vi "Run In UI.vi"(11 "LUnit Test Case in":refnum<class "LUnit Test Case.lvclass">) -> (3 "LUnit Test Case out":refnum<class "LUnit Test Case.lvclass">)   [LabVIEW 2020, in "LUnit Test Case.lvclass"]
uses:
  LUnit Test Case.lvclass
  LUnit Test Case.lvclass/LUnit Test Case.ctl
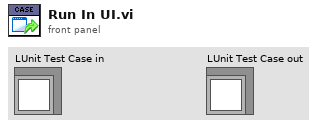
[diagram p1: front panel]
types:
  T1 = enum32{"Invalid", "Standard", "Closed", "Hidden", "Minimized", "Maximized"}
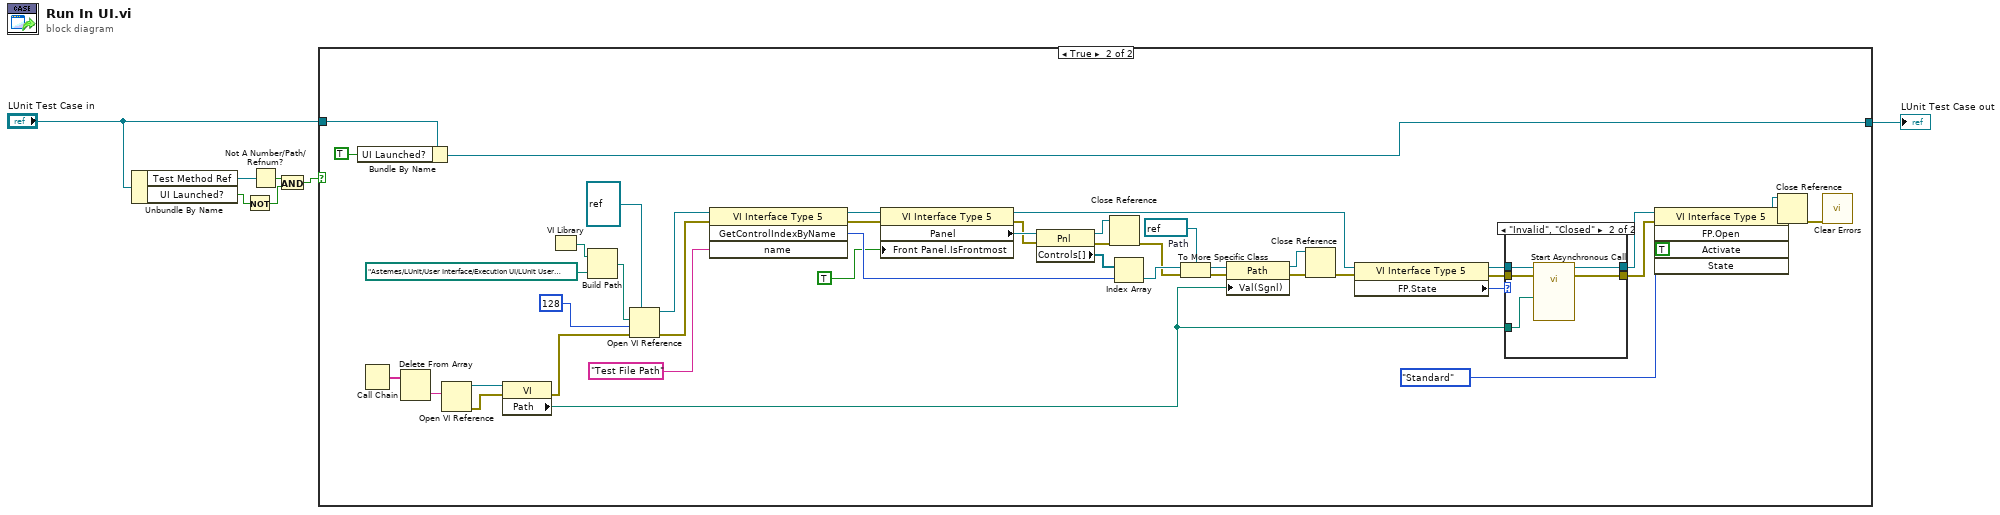
[diagram p0: block diagram]
diagram:
  n1 = Unbundle By Name("LUnit Test Case in") -> ("Test Method Ref"=w7:refnum<vi>, "UI Launched?"=w4:bool)
  n2 = Not(x=w4) -> (.not. x?=w3:bool)
  n3 = Not A Number/Path/Refnum?(number/path/refnum=w7) -> (NaN/Path/Refnum?=w6:bool)
  n4 = And(x=w6, y=w3) -> (x .and. y?=w5:bool)
  n5 = case shown="True" w5 {
    tunnel: "LUnit Test Case in" -> [w8 w11]
    tunnel: [w8 w9] -> w1
    frame False {
    }
    frame True {
      w40 = refnum<vi> refnum  # Path
      n6 = Bundle By Name(cluster=w11, "UI Launched?"=TRUE) -> (w9:refnum<class "LUnit Test Case.lvclass">)
      n7 = Call Chain() -> (call chain=w13:string[])
      n8 = Delete From Array(array=w13) -> (deleted portion=w17:string)  [unwired: 2 in, 1 out]
      n9 = Open VI Reference(vi path=w17) -> (vi reference=w16:refnum<vi>, error out=w14:errorcluster)  [unwired: 5 in]
      n10 = property class="VI"(reference=w16, error in=w14) -> (error out=w15:errorcluster, "Path"=w12:path)  [unwired: 1 out]
      n11 = VI Library() -> (path=w46:path)
      n12 = Build Path(base path=w46, name or relative path=path "Astemes/LUnit/User Interface/Execution UI/LUnit User Interface.vi" ("Relative Path from 1 to 2")) -> (appended path=w51:path)
      n13 = Open VI Reference(type specifier VI Refnum (for type only)=refnum<vi> refnum, vi path=w51, options=128, error in (no error)=w15) -> (vi reference=w28:refnum<vi>, error out=w27:errorcluster)  [unwired: 2 in]
      n14 = invoke class="VI Interface Type 5" method="GetControlIndexByName"(reference=w28, error in=w27, "name"="Test File Path" ("Control Name")) -> (reference out=w44:refnum<vi>, error out=w34:errorcluster, "GetControlIndexByName"=w41:i32)  [unwired: 1 in, 1 out]
      n15 = property class="VI Interface Type 5"(reference=w44, error in=w34, "Front Panel.IsFrontmost"=TRUE ("Front Panel Window:Is Frontmost")) -> (reference out=w21:refnum<vi>, error out=w35:errorcluster, "Panel"=w45:refnum<vi>)
      n16 = property class="Pnl"(reference=w45, error in=w35) -> (reference out=w31:refnum<vi>, error out=w36:errorcluster, "Controls[]"=w42:refnum<vi>[])
      n17 = Close Reference(reference=w31, error in (no error)=w36) -> (error out=w32:errorcluster)
      n18 = Index Array(array=w42, index=w41) -> (element=w38:refnum<vi>)
      n19 = To More Specific Class(target class=w40, reference=w38, error in=w32) -> (specific class reference=w39:refnum<vi>, error out=w37:errorcluster)
      n20 = property class="Path"(reference=w39, error in=w37, "Val(Sgnl)"=w12) -> (reference out=w30:refnum<vi>, error out=w33:errorcluster)
      n21 = Close Reference(reference=w30, error in (no error)=w33) -> (error out=w23:errorcluster)
      n22 = property class="VI Interface Type 5"(reference=w21, error in=w23) -> (reference out=w25:refnum<vi>, error out=w26:errorcluster, "FP.State"=w24:T1)
      n23 = case shown="\"Invalid\", \"Closed\"" w24 {
        tunnel: w26 -> [w55 w60]
        tunnel: w25 -> [w54 w59]
        tunnel: [w55 w57] -> w22
        tunnel: [w54 w58] -> w20
        tunnel: w12 -> [_ w56]
        frame Default {
        }
        frame "Invalid", "Closed" {
          n24 = call-by-ref "Start Asynchronous Call"(reference=w59, error in=w60, "Test File Path"=w56) -> (reference out=w58:refnum<vi>, error out=w57:errorcluster)  [unwired: 11 in]
        }
      }
      n25 = invoke class="VI Interface Type 5" method="FP.Open"(reference=w20, error in=w22, "Activate"=TRUE ("Activate?"), "State"=T1."Standard") -> (reference out=w50:refnum<vi>, error out=w49:errorcluster)  [unwired: 1 in, 3 out]
      n26 = Close Reference(reference=w50, error in (no error)=w49) -> (error out=w19:errorcluster)
      n27 = call <vilib>:"Clear Errors.vi"("error in (no error)"=w19) -> ()  [unwired: 5 in, 2 out]
    }
  }
  "LUnit Test Case out" <- w1
